vi "ReadHeliumMonitorCfg.vi"(7 "section":string="General", 8 "Error In":errorcluster, 10 "Sensors":T1[](array[typedef])=[{"Name"="Ghz lab", "URL"="http:\\\\130.55.69.25", "Channels"=[{"type"=enum."Flow meter", "number"=6.0}]}, {"Name"="main bag", "URL"="http:\\\\130.55.69.22", "Channels"=[{"type"=enum."Flow meter", "number"=6.0}, {"type"=enum."Tank pressure", "number"=0.0}, {"type"=enum."Dewar level", "number"=1.0}]}, {"Name"="PPMS 20T", "URL"="http:\\\\130.55.69.42", "Channels"=[{"type"=enum."Flow meter", "number"=6.0}]}], 11 "CFG File Path":path) -> (0 "Error Out":errorcluster, 2 "Sensors out":T1[](array[typedef])=[{"Name"="Ghz lab", "URL"="http:\\\\130.55.69.25", "Channels"=[{"type"=enum."Flow meter", "number"=6.0}]}, {"Name"="main bag", "URL"="http:\\\\130.55.69.22", "Channels"=[{"type"=enum."Flow meter", "number"=6.0}, {"type"=enum."Tank pressure", "number"=0.0}, {"type"=enum."Dewar level", "number"=1.0}]}, {"Name"="PPMS 20T", "URL"="http:\\\\130.55.69.42", "Channels"=[{"type"=enum."Flow meter", "number"=6.0}]}], 3 "CFG File Path out":path)   [LabVIEW 2015]
uses:
  Sensor configuration.ctl
  Channel type.ctl
  <vilib>/Utility/config.llb/NI_LVConfig.lvlib
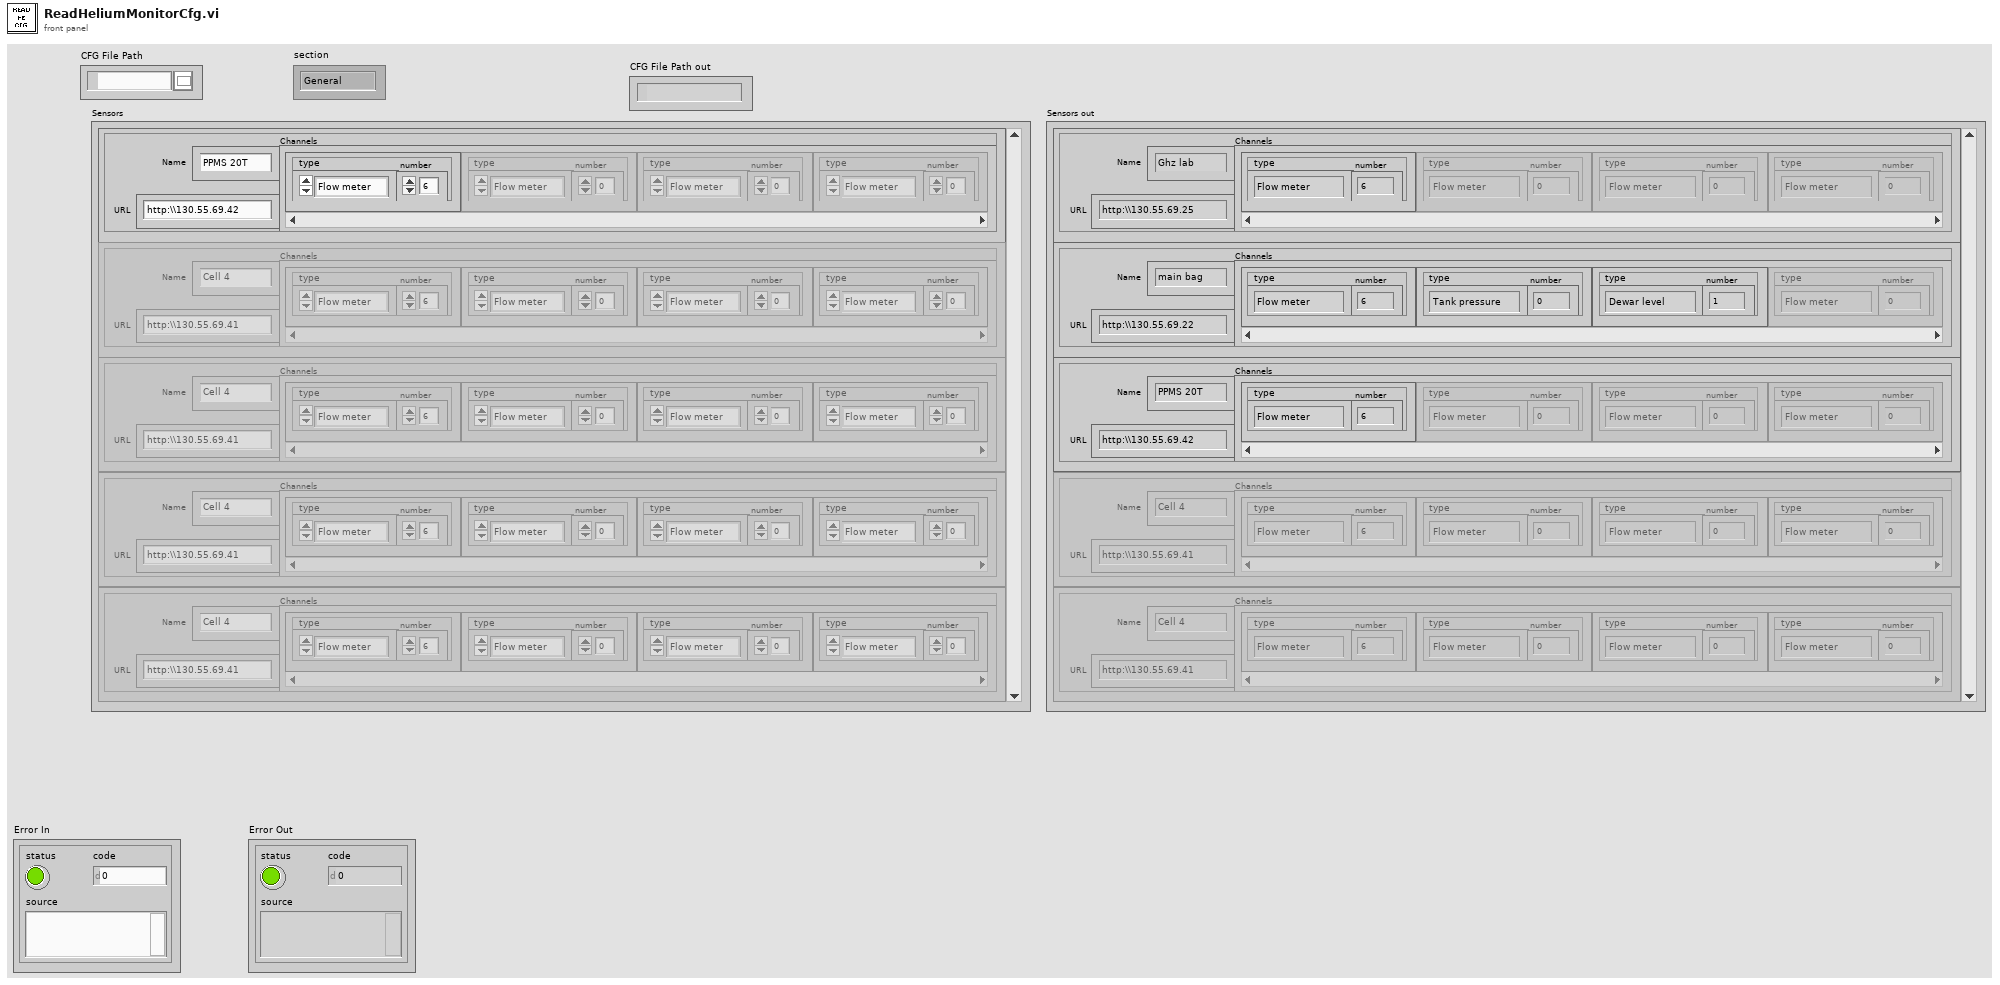
[diagram p1: front panel]
types:
  T1 = typedef "Sensor configuration.ctl" = cluster{"Name":string, "URL":string, "Channels":cluster{"type":T2, "number":dbl}[]}
  T2 = typedef "Channel type.ctl" = enum16{"Volts", "Flow meter", "Tank pressure", "Dewar level", "Raw ADC"}
  T3 = typedef "NI_LVConfig.lvlib/Config Data RefNum.ctl" = refnum<k1>
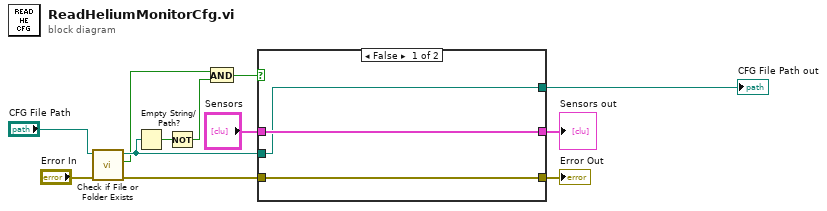
[diagram p0: block diagram]
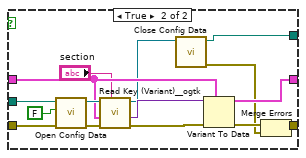
[diagram p2: hidden frame]
diagram:
  n1 = call <vilib>:"Check if File or Folder Exists.vi"("error in (no error)"="Error In", "path"="CFG File Path") -> ("error out"=w7:errorcluster, "file or folder exists?"=w5:bool, "dup path"=w11:path)  [unwired: 7 in]
  n2 = Empty String/Path?(string/path=w11) -> (empty?=w10:bool)
  n3 = Not(x=w10) -> (.not. x?=w4:bool)
  n4 = And(x=w5, y=w4) -> (x .and. y?=w3:bool)
  n5 = case shown="False" w3 {
    tunnel: w11 -> [w13 w28]
    tunnel: "Sensors" -> [w14 w22]
    tunnel: w7 -> [w15 w27]
    tunnel: [w15 w18] -> w6
    tunnel: [w14 w23] -> w2
    tunnel: [w13 w16] -> w1
    frame False {
    }
    frame True {
      n6 = call <vilib>:"Open Config Data.vi"("error in (no error)"=w27, "create file if necessary (T)"=FALSE, "configuration file path"=w28) -> ("error out"=w26:errorcluster, "refnum"=w30:T3)  [unwired: 6 in, 1 out]
      n7 = call <userlib>:"Read Key (Variant)__ogtk.vi"("section"="section", "error in (no error)"=w26, "type"=w22, "refnum"=w30) -> ("error out"=w25:errorcluster, "key-value"=w21:variant, "refnum out"=w19:T3)  [unwired: 4 in, 1 out]
      n8 = call <vilib>:"Close Config Data.vi"("refnum"=w19) -> ("error out"=w17:errorcluster, "file path"=w16:path)  [unwired: 9 in]
      n9 = Variant To Data(error in=w25, type=w22, Variant=w21) -> (data=w23:T1[], error out=w24:errorcluster)
      n10 = Merge Errors(w24, w17) -> (w18:errorcluster)
    }
  }
  "Error Out" <- w6
  "Sensors out" <- w2
  "CFG File Path out" <- w1
